vi "Ctor.vi"(8 "error in (no error)":errorcluster, 11 "WebSocket Ref":refnum<data-value>) -> (0 "error out":errorcluster, 3 "WebSocket Handler out":refnum<class "WebSocket Handler.lvclass">)   [LabVIEW 2020, in "HTTP Server.lvlib" / "WebSocket Handler.lvclass"]
uses:
  WebSocket Handler.lvclass
  WebSocket Data.ctl
  WebSocket Manager/WebSocket Manager.lvclass
  WebSocket Handler.lvclass/WebSocket Handler.ctl
  HTTP Server.lvlib
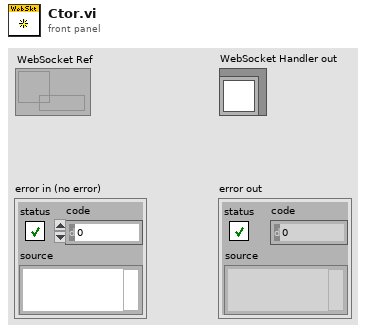
[diagram p1: front panel]
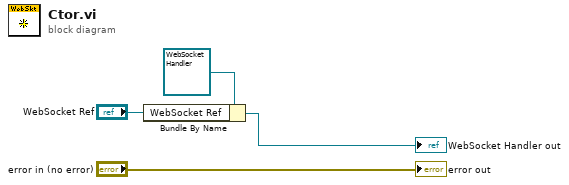
[diagram p0: block diagram]
diagram:
  n1 = Bundle By Name(cluster=refnum<class "WebSocket Handler.lvclass"> refnum ("WebSocket Handler in"), "WebSocket Ref"="WebSocket Ref") -> (→"WebSocket Handler out":refnum<class "WebSocket Handler.lvclass">)
  "error out" <- "error in (no error)"
